vi "Image-RGB to I16 conversion.vi"(8 "error in (no error)":errorcluster, 10 "I16 image ref in":T1, 11 "RGB image ref in":T1) -> (0 "error out":errorcluster, 3 "I16 image ref out":T1)   [LabVIEW 2017]
uses:
  <vilib>/vision/Image Controls.llb/IMAQ Image.ctl
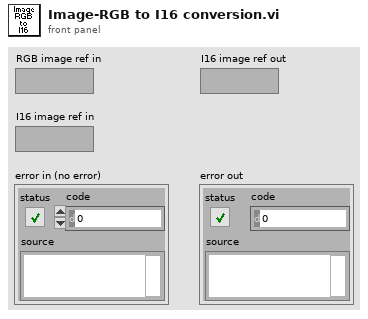
[diagram p1: front panel]
types:
  T1 = typedef "IMAQ Image.ctl" = refnum<image>
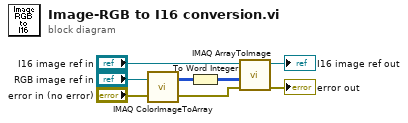
[diagram p0: block diagram]
diagram:
  n1 = call "IMAQ ColorImageToArray"("Image"="RGB image ref in", "error in (no error)"="error in (no error)") -> ("Image Pixels (U32)"=w4:u32[][], "error out"=w8:errorcluster)  [unwired: 1 in, 2 out]
  n2 = To Word Integer(number=w4) -> (16bit integer=w1:i16[][])
  n3 = call "IMAQ ArrayToImage"("error in (no error)"=w8, "Image Pixels (I16)"=w1, "Image"="I16 image ref in") -> ("error out"=→"error out":errorcluster, "Image Out"=→"I16 image ref out":T1)  [unwired: 7 in]
